vi "Create Grayscale image.vi"(10 "image data":T1) -> (2 "Gray scale Image":T1)   [LabVIEW 2012, in "Button.lvclass"]
doc: "Converts a flattened image into a grey scale image. This is used to generate a disabled button image from a colour image"
uses:
  Button.lvclass
  <vilib>/picture/picture.llb/imagedata.ctl
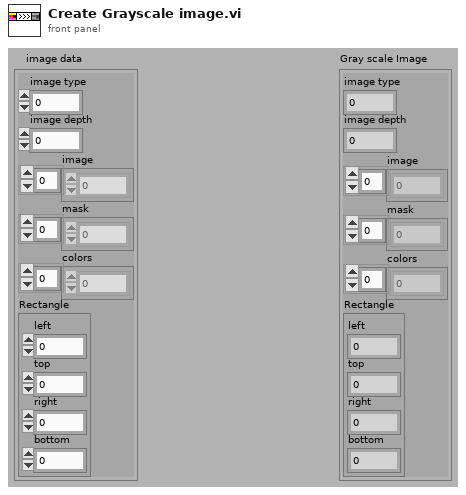
[diagram p1: front panel]
types:
  T1 = typedef "imagedata.ctl" = cluster{"image type":i32, "image depth":i32, "image":u8[], "mask":u8[], "colors":u32[], "Rectangle":cluster{"left":i16, "top":i16, "right":i16, "bottom":i16}}
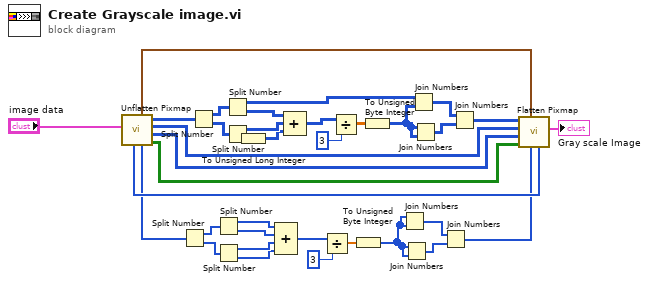
[diagram p0: block diagram]
diagram:
  n1 = call <vilib>:"Unflatten Pixmap.vi"("image data"="image data") -> ("1-bit pixmap"=w20:bool[][], "4-bit pixmap"=w21:u8[][], "8-bit pixmap"=w22:u8[][], "24-bit pixmap"=w35:u32[][], "colors"=w8:u32[], "top left"=w6:cluster{"x":i16, "y":i16}, "mask"=w19:u8[])  [unwired: 4 out]
  n2 = Split Number(x=w8) -> (hi(x)=w9:u16[], lo(x)=w10:u16[])
  n3 = Split Number(x=w35) -> (hi(x)=w34:u16[][], lo(x)=w33:u16[][])
  n4 = Split Number(x=w9) -> (hi(x)=w11:u8[], lo(x)=w12:u8[])
  n5 = Split Number(x=w10) -> (hi(x)=w13:u8[], lo(x)=w4:u8[])
  n6 = Split Number(x=w34) -> (hi(x)=w1:u8[][], lo(x)=w32:u8[][])
  n7 = Split Number(x=w33) -> (hi(x)=w31:u8[][], lo(x)=w30:u8[][])
  n8 = To Unsigned Long Integer(number=w30) -> (unsigned 32bit integer=w2:u32[][])
  n9 = Compound Arithmetic op=ADD(w11, w12, w13, w4) -> (w14:u8[])
  n10 = Compound Arithmetic op=ADD(w32, w31, w2) -> (w29:u32[][])
  n11 = Divide(x=w14, y=3) -> (x/y=w15:dbl[])
  n12 = Divide(x=w29, y=3) -> (x/y=w27:dbl[][])
  n13 = To Unsigned Byte Integer(number=w15) -> (unsigned 8bit integer=w18:u8[])
  n14 = To Unsigned Byte Integer(number=w27) -> (unsigned 8bit integer=w24:u8[][])
  n15 = Join Numbers(hi=w18, lo=w18) -> ((hi.lo)=w17:u16[])
  n16 = Join Numbers(hi=w18, lo=w18) -> ((hi.lo)=w16:u16[])
  n17 = Join Numbers(hi=w1, lo=w24) -> ((hi.lo)=w25:u16[][])
  n18 = Join Numbers(hi=w24, lo=w24) -> ((hi.lo)=w26:u16[][])
  n19 = Join Numbers(hi=w17, lo=w16) -> ((hi.lo)=w7:u32[])
  n20 = Join Numbers(hi=w25, lo=w26) -> ((hi.lo)=w23:u32[][])
  n21 = call <vilib>:"Flatten Pixmap.vi"("mask"=w19, "colors"=w7, "top left"=w6, "1-bit pixmap"=w20, "4-bit pixmap"=w21, "8-bit pixmap"=w22, "24-bit pixmap"=w23) -> ("image data"=→"Gray scale Image":T1)  [unwired: 4 out]
